vi "009 Circumferència mod.vi"() -> ()   [LabVIEW 2019]
panel:
  in  "stop":bool
  in  "Numeric":dbl
  out "XY Graph":cluster{dbl[], dbl[]}(graph)
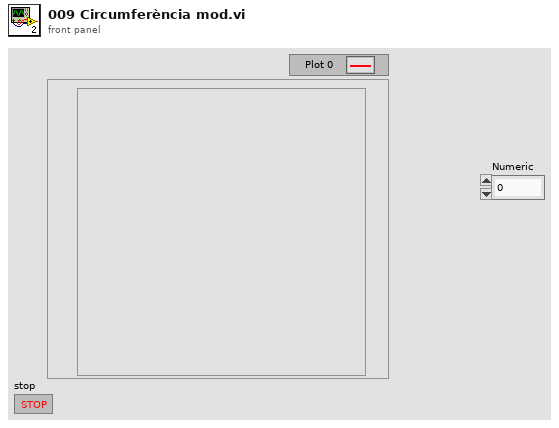
[diagram p1: front panel]
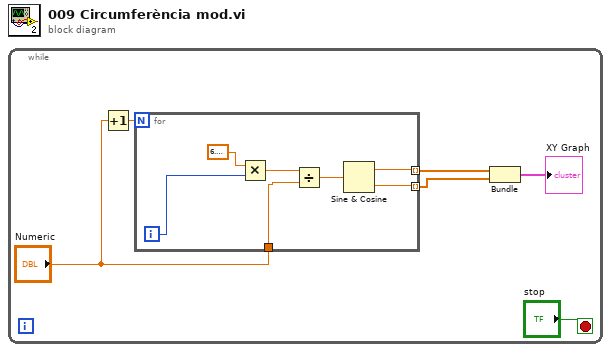
[diagram p0: block diagram]
diagram:
  n1 = while {
    stop <- "stop" stop-if-true
    n2 = Increment(x="Numeric") -> (x+1=w3:dbl)
    n3 = for {
      N: w3 -> [_]
      tunnel: [w9] -> w5 mode=indexing
      tunnel: [w8] -> w4 mode=indexing
      tunnel: "Numeric" -> [w7]
      i -> [w13]
      n4 = Multiply(x=6.283185307179586, y=w13) -> (x*y=w11:dbl)
      n5 = Divide(x=w11, y=w7) -> (x/y=w10:dbl)
      n6 = Sine & Cosine(0:w10) -> (1:w9:dbl, 2:w8:dbl)
    }
    n7 = Bundle(w5, w4) -> (→"XY Graph":cluster{dbl[], dbl[]})  [unwired: 1 in]
  }
